vi "Change Speaker Waveform.vi"(8 "error in":errorcluster, 11 "cPAS in":refnum<class "cPAS.lvclass">) -> (0 "error out":errorcluster, 3 "cPAS out":refnum<class "cPAS.lvclass">)   [LabVIEW 2015, in "cPAS.lvclass"]
doc: "Check shared variables f_cent and Df to generate a new chirp signal. f_cent is intended to be the center frequency of the chirp and Df is the full bandwidth of the chirp.\n\nThe VI calls Init Tophat LUT - tophat refers to the signal shape in the frequency domain."
uses:
  cPAS.lvclass
  Reusable/PAS/Main/PAS.lvclass/PAS.ctl
  cPAS.lvclass/cPAS.ctl
  Reusable/PAS/Main/Write Chirp.vi
  <vilib>/Utility/error.llb/Error Cluster From Error Code.vi
  <vilib>/rvi/errors/niLvFpgaAdjustHostInterfaceError.vi
  <vilib>/rvi/interface/nirviMethod/nirviMethod.xnode
  Interface/fpga_ctl.ctl
  FPGA Bitfiles/FPGA Server.lvbitx
  <vilib>/FPGAPlugInAG/PXI-7841R/niLvFpga_WriteFifo_PXI-7841R.vi
  <vilib>/rvi/errors/niLvFpgaMergeErrorWithErrorCode.vi
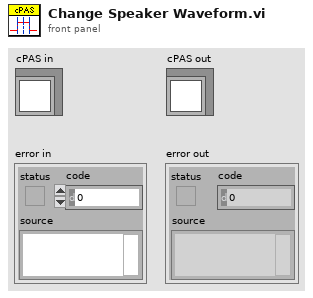
[diagram p1: front panel]
types:
  T1 = typedef "fpga_ctl.ctl" = refnum<k20>
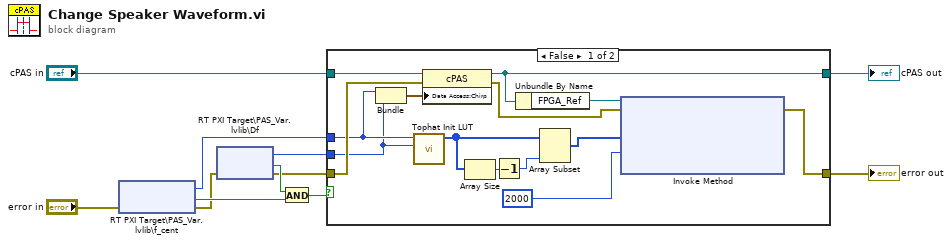
[diagram p0: block diagram]
diagram:
  n1 = shared-variable "RT PXI Target\\PAS_Var.lvlib\\f_cent"(error in="error in") -> (w7:i16, error out=w4:errorcluster, w10:bool)  [unwired: 1 in]
  n2 = shared-variable "RT PXI Target\\PAS_Var.lvlib\\Df"(error in=w4) -> (w8:i16, error out=w3:errorcluster, w11:bool)  [unwired: 1 in]
  n3 = And(x=w11, y=w10) -> (x .and. y?=w9:bool)
  n4 = case shown="False" w9 {
    tunnel: w8 -> [w17 _]
    tunnel: w7 -> [w18 _]
    tunnel: "cPAS in" -> [w22 w27]
    tunnel: [w21 w27] -> w6
    tunnel: w3 -> [w20 w26]
    tunnel: [w23 w26] -> w2
    frame False {
      n5 = Bundle("Int16"=w18, "Int16"=w17) -> (w16:cluster{"Int16":i16, "Int16":i16})  [unwired: 1 in]
      n6 = call "Tophat Init LUT.vi"("Df"=w17, "f0"=w18) -> ("Init Data Out"=w15:i16[])  [unwired: 7 in]
      n7 = property class="cPAS"(reference=w22, error in=w20, "Data Access:Chirp"=w16) -> (reference out=w21:refnum<class "cPAS.lvclass">, error out=w19:errorcluster)
      n8 = Array Size(array=w15) -> (size(s)=w14:i32)
      n9 = Decrement(x=w14) -> (x-1=w13:i32)
      n10 = Unbundle By Name(w21) -> ("FPGA_Ref"=w25:T1)
      n11 = Array Subset(array=w15, length=w13) -> (w12:i16[])  [unwired: 1 in]
      n12 = xnode "Invoke Method"("FPGA VI Reference In"=w25, "error in"=w19, "Data"=w12, "Timeout (ms)"=2000) -> ("error out"=w23:errorcluster)  [unwired: 2 out]
    }
    frame True {
    }
  }
  "error out" <- w2
  "cPAS out" <- w6
